vi "Allarmi_High_Low_Field.vi"(1 "Numeric":dbl, 4 "Ripetizioni alarm Hf":bool, 5 "reference 5":refnum<vi>, 6 "reference 4":refnum<vi>, 7 "reference 3":refnum<vi>, 8 "Ripetizioni alarm VHf":bool, 9 "reference 2":refnum<vi>, 10 "reference":refnum<vi>) -> (0 "String Alarm":string, 2 "In allarme VHf ?":bool, 3 "In allarme Hf ?":bool)   [LabVIEW 2010]
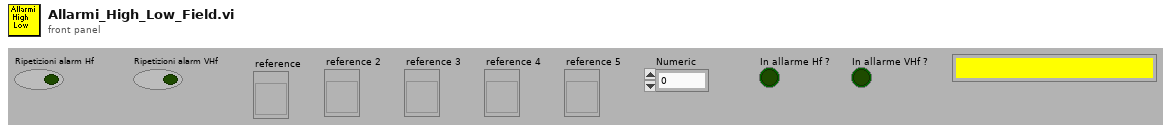
[diagram p1: front panel]
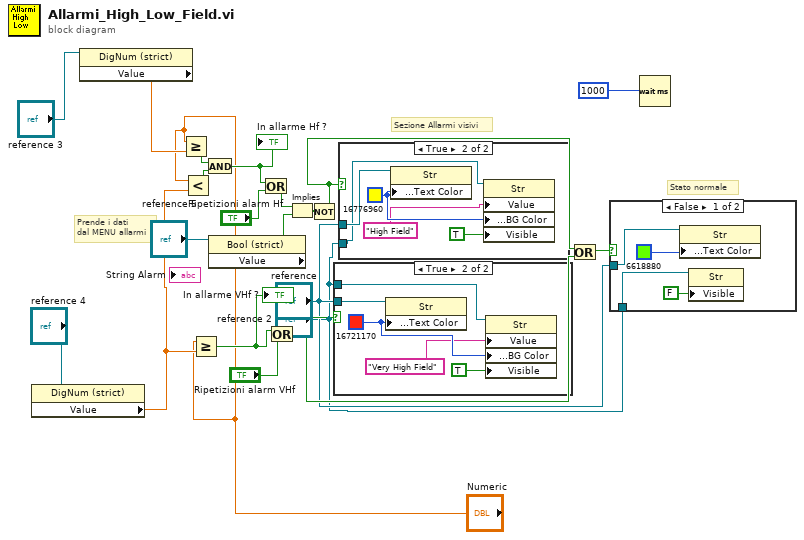
[diagram p0: block diagram]
diagram:
  # "Prende i dati\ndal MENU allarmi"
  # "Stato normale"
  # "Sezione Allarmi visivi"
  n1 = property on="Property Node" class="DigNum (strict)"(reference="reference 4") -> ("Value"=w11:sgl)  [unwired: 1 in, 2 out]
  n2 = property on="Property Node" class="DigNum (strict)"(reference="reference 3") -> ("Value"=w10:sgl)  [unwired: 1 in, 2 out]
  n3 = Greater Or Equal?(x="Numeric", y=w10) -> (x >= y?=w8:bool)
  n4 = Less?(x="Numeric", y=w11) -> (x < y?=w9:bool)
  n5 = Greater Or Equal?(x="Numeric", y=w11) -> (x >= y?=w14:bool)
  "In allarme VHf ?" <- w14
  n6 = And(x=w8, y=w9) -> (x .and. y?=w13:bool)
  "In allarme Hf ?" <- w13
  n7 = property on="Property Node" class="Bool (strict)"(reference="reference 5") -> ("Value"=w19:bool)  [unwired: 1 in, 2 out]
  n8 = Or(x=w13, y="Ripetizioni alarm Hf") -> (x .or. y?=w18:bool)
  n9 = Or(x=w14, y="Ripetizioni alarm VHf") -> (x .or. y?=w17:bool)
  n10 = Implies(1:w19, 2:w18) -> (0:w20:bool)
  n11 = Not(x=w20) -> (.not. x?=w21:bool)
  n12 = case shown="True" w17 {
    tunnel: "reference" -> [_ w23]
    tunnel: "reference 2" -> [_ w22]
    frame False {
    }
    frame True {
      w25 = u32 16721170
      n13 = property on="Property Node" class="Str"(reference=w23, "Text.Text Colors:Text Color"=w25) -> ()  [unwired: 1 in, 2 out]
      n14 = property on="Property Node" class="Str"(reference=w22, "Value"="Very High Field", "Text.Text Colors:BG Color"=w25, "Visible"=TRUE) -> ()  [unwired: 1 in, 2 out]
    }
  }
  n15 = case shown="True" w21 {
    tunnel: "reference" -> [_ w28]
    tunnel: "reference 2" -> [_ w27]
    frame False {
    }
    frame True {
      w31 = u32 16776960
      n16 = property on="Property Node" class="Str"(reference=w28, "Text.Text Colors:Text Color"=w31) -> ()  [unwired: 1 in, 2 out]
      n17 = property on="Property Node" class="Str"(reference=w27, "Value"="High Field", "Text.Text Colors:BG Color"=w31, "Visible"=TRUE) -> ()  [unwired: 1 in, 2 out]
    }
  }
  n18 = Or(x=w21, y=w17) -> (x .or. y?=w16:bool)
  n19 = case shown="False" w16 {
    tunnel: "reference" -> [w33 _]
    tunnel: "reference 2" -> [w32 _]
    frame False {
      n20 = property on="Property Node" class="Str"(reference=w33, "Text.Text Colors:Text Color"=u32 6618880) -> ()  [unwired: 1 in, 2 out]
      n21 = property on="Property Node" class="Str"(reference=w32, "Visible"=FALSE) -> ()  [unwired: 1 in, 2 out]
    }
    frame True {
    }
  }
  n22 = Wait (ms)(milliseconds to wait=1000) -> ()  [unwired: 1 out]
